vi "SMBUS Init.vi"(7 "EnablePu":u8, 9 "ClockSpeedHz":i32, 10 "IICIndex":i32, 11 "DevIndex":i32) -> (3 "function return":i32)   [LabVIEW 2010, in "usb2iic.lvlib"]
doc: "int WINAPI SMBUS_Init(int DevIndex,int IICIndex,int ClockSpeedHz,unsigned char EnablePu);"
uses:
  usb2iic.lvlib
  USB2XXX.dll
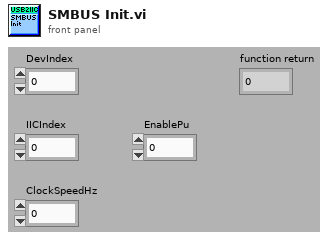
[diagram p1: front panel]
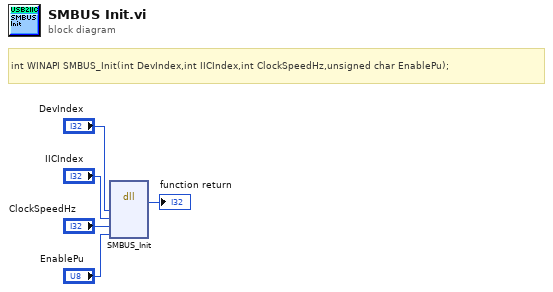
[diagram p0: block diagram]
diagram:
  # "int WINAPI SMBUS_Init(int DevIndex,int IICIndex,int ClockSpeedHz,unsigned char EnablePu);"
  n1 = dll-call lib="G:/OtherWork/USB2XXX_Example/trunk/Labview/PublicFiles/usb2iic/USB2XXX.*" fn="SMBUS_Init"("DevIndex"="DevIndex", "IICIndex"="IICIndex", "ClockSpeedHz"="ClockSpeedHz", "EnablePu"="EnablePu") -> (→"function return":i32)  [unwired: 7 in, 2 out]
